vi "Set Result Name.vi"(8 "error in (no error)":errorcluster, 10 "Step In":refnum<k7>, 11 "Skyworks - PVT in":refnum<class "Skyworks - PVT.lvclass">) -> (0 "error out":errorcluster, 2 "Step Out":refnum<k7>, 3 "Skyworks - PVT out":refnum<class "Skyworks - PVT.lvclass">)   [LabVIEW 2018, in "Skyworks PVT.lvlib" / "Skyworks - PVT.lvclass"]
uses:
  Skyworks - PVT.lvclass
  C:/Sequence Automation/Plugins/Measurement Interface.lvlibp/Measurement Interface.lvclass
  Plugins/Measurement Interface.lvlibp/Private Methods/Measurement Name/Read Measurement Name.vi
  Plugins/TestStand API Tools (TSAT).lvlibp/Step Actions/TSAT Step Actions.lvlib
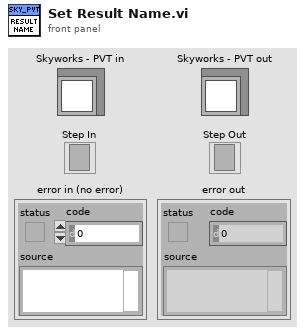
[diagram p1: front panel]
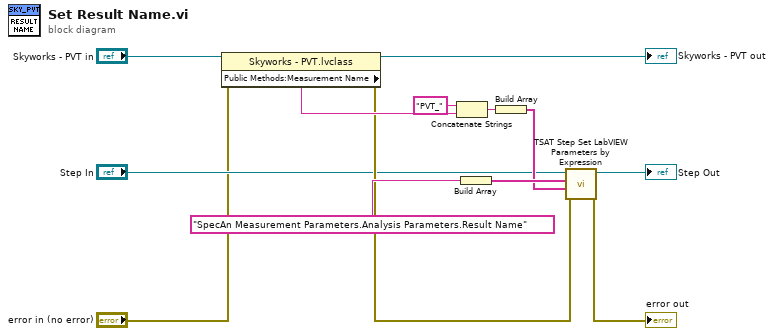
[diagram p0: block diagram]
diagram:
  n1 = property class="Skyworks - PVT.lvclass"(reference="Skyworks - PVT in", error in="error in (no error)") -> (reference out=→"Skyworks - PVT out":refnum<class "Skyworks - PVT.lvclass">, error out=w7:errorcluster, "Public Methods:Measurement Name"=w11:string)
  n2 = Concatenate Strings("PVT_" ("string"), w11) -> (w9:string)
  n3 = Build Array("SpecAn Measurement Parameters.Analysis Parameters.Result Name") -> (w12:string[])
  n4 = Build Array(w9) -> (w8:string[])
  n5 = call "TSAT Step Set LabVIEW Parameters by Expression.vi"("Error In"=w7, "Value Expressions"=w8, "Parameters to Set"=w12, "Step In"="Step In") -> ("Error Out"=→"error out":errorcluster, "Step Out"=→"Step Out":refnum<k7>)  [unwired: 6 in]
